vi "DeviceToSize.vi"(8 "error in (no error)":errorcluster, 11 "DeviceType in":u16) -> (0 "error out":errorcluster, 3 "Size":u16)   [LabVIEW 2015]
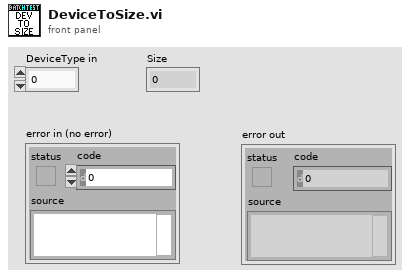
[diagram p1: front panel]
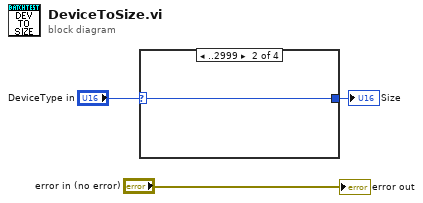
[diagram p0: block diagram]
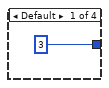
[diagram p2: hidden frame]
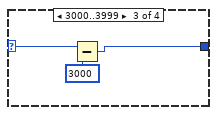
[diagram p3: hidden frame]
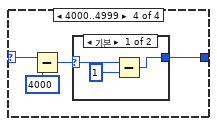
[diagram p4: hidden frame]
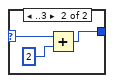
[diagram p5: hidden frame]
diagram:
  n1 = case shown="..2999" "DeviceType in" {
    selector: "DeviceType in" -> [_ w5 w8 w12]
    tunnel: [u16 3 w5 w7 w9] -> w3
    frame Default {
    }
    frame ..2999 {
    }
    frame 3000..3999 {
      n2 = Subtract(x=w8, y=u16 3000) -> (x-y=w7:u16)
    }
    frame 4000..4999 {
      n3 = Subtract(x=w12, y=u16 4000) -> (x-y=w10:u16)
      n4 = case shown="기본" w10 {
        selector: w10 -> [w15 w18]
        tunnel: [w14 w17] -> w9
        frame Default {
          n5 = Subtract(x=w15, y=u16 1) -> (x-y=w14:u16)
        }
        frame ..3 {
          n6 = Add(x=w18, y=u16 2) -> (x+y=w17:u16)
        }
      }
    }
  }
  "Size" <- w3
  "error out" <- "error in (no error)"
